vi "Track Loop Rate.vi"(10 "Refresh Rate":i32) -> (1 "Late Count":i32, 2 "Loop Time":u32, 3 "Late?":bool)   [LabVIEW 2020, in "Modbus Master Engine.lvlib"]
uses:
  Modbus Master Engine.lvlib
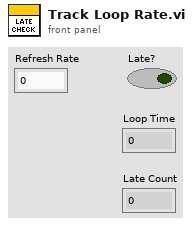
[diagram p1: front panel]
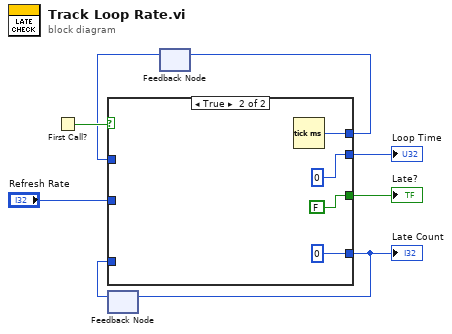
[diagram p0: block diagram]
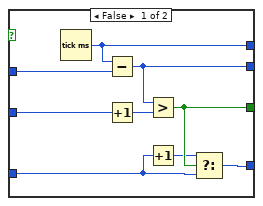
[diagram p2: hidden frame]
diagram:
  n1 = First Call?() -> (First Call?: T/F=w8:bool)
  n2 = feedback #1() -> (w2:i32)  [unwired: 1 in]
  n3 = feedback #2() -> (w6:u32)  [unwired: 1 in]
  n4 = case shown="True" w8 {
    tunnel: [w16 w21] -> w7
    tunnel: w6 -> [w17 _]
    tunnel: "Refresh Rate" -> [w11 _]
    tunnel: [w15 FALSE] -> w4
    tunnel: [w12 0] -> w3
    tunnel: w2 -> [w14 _]
    tunnel: [w9 u32 0] -> w1
    frame False {
      n5 = Tick Count (ms)() -> (millisecond timer value=w16:u32)
      n6 = Subtract(x=w16, y=w17) -> (x-y=w9:u32)
      n7 = Increment(x=w11) -> (x+1=w10:i32)
      n8 = Greater?(x=w9, y=w10) -> (0:w15:bool)
      n9 = Increment(x=w14) -> (x+1=w13:i32)
      n10 = Select(t=w13, s=w15, f=w14) -> (s? t:f=w12:i32)
    }
    frame True {
      n11 = Tick Count (ms)() -> (millisecond timer value=w21:u32)
    }
  }
  "Late?" <- w4
  "Late Count" <- w3
  "Loop Time" <- w1
  n12 = feedback-in #1(w3) -> ()
  n13 = feedback-in #2(w7) -> ()
